vi "Get Ethernet Port.vi"(8 "Error In":errorcluster, 11 "LINX Device Config":T1) -> (0 "Error Out":errorcluster, 2 "Ethernet Port":u16, 3 "LINX Device Config":T1)   [LabVIEW 2020, in "LMH-LINX.lvlib" / "Device.lvlib"]
doc: "Get the LINX device's Ethernet Port."
uses:
  Device.lvlib
  Type Defs/LINX Device Config.ctl
  Type Defs/Interface.ctl
  Type Defs/TCP Config.ctl
  Type Defs/Channels.ctl
  Type Defs/Error Type.ctl
  LMH-LINX.lvlib
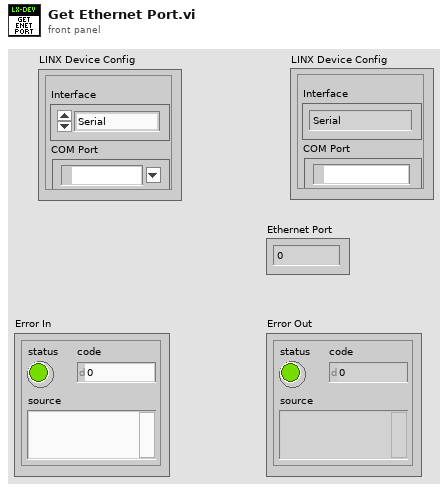
[diagram p1: front panel]
types:
  T1 = typedef "LMH-LINX.lvlib/Device.lvlib/LINX Device Config.ctl" = cluster{"Interface":T2, "COM Port":refnum<visa-resource-name>, "TCP Configuration":T3, "Device Family":u8, "Device ID":u8, "Device Name":string, "TCP Ref":refnum<k5>, "Channels":T4}
  T2 = typedef "LMH-LINX.lvlib/Interface.ctl" = enum16{"Serial", "TCP"}
  T3 = typedef "LMH-LINX.lvlib/Device.lvlib/TCP Config.ctl" = cluster{"IP Address":string, "Port":u16}
  T4 = typedef "LMH-LINX.lvlib/Channels.ctl" = cluster{"DI":u8[], "DO":u8[], "AI":u8[], "AO":u8[], "PWM":u8[], "QE":u8[], "UART":u8[], "I2C 2":u8[], "SPI":u8[], "CAN":u8[], "Servo":u8[], "AI Ref (V)":dbl, "AI Resolution (Bits)":u8, "AO Ref (V)":dbl, "AO Resolution (Bits)":u8}
  T5 = typedef "LMH-LINX.lvlib/Error Type.ctl" = enum16{"Unknown", "Timeout", "Corrupt Return Packet", "Unable To Connect", "Command Not Supported", "Channel DNE", "Invalid COM Config", "Firmware Version Mismatch", "myRIO Support", "CMD Specific Error", "Local IO Not Supported"}
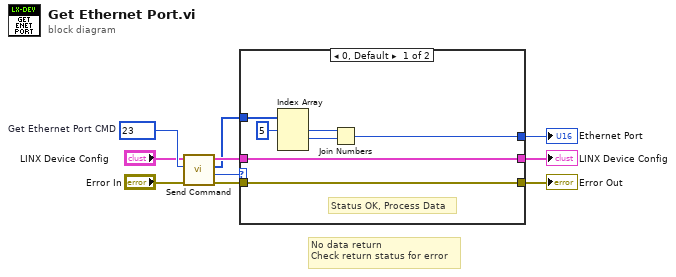
[diagram p0: block diagram]
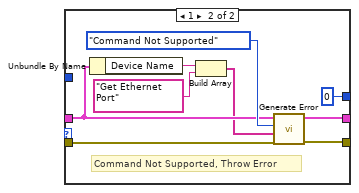
[diagram p2: hidden frame]
diagram:
  w9 = u16 23  # Get Ethernet Port CMD
  # "No data return\nCheck return status for error"
  n1 = call "Send Command.vi"("Error In"="Error In", "CMD"=w9, "LINX Device Config"="LINX Device Config") -> ("Error Out"=w4:errorcluster, "Status"=w1:u8, "Response"=w3:u8[], "LINX Device Config"=w6:T1)  [unwired: 5 in]
  n2 = case shown="0, Default" w1 {
    tunnel: [w16 w24] -> w7
    tunnel: w6 -> [w16 w20]
    tunnel: [w17 w25] -> w5
    tunnel: w4 -> [w17 w26]
    tunnel: w3 -> [w15 _]
    tunnel: [w11 u16 0] -> w2
    frame 0, Default {
      # "Status OK, Process Data"
      n3 = Index Array(array=w15, index #1=5 ("index")) -> (element #1=w13:u8, element #2=w12:u8)  [unwired: 2 in, 1 out]
      n4 = Join Numbers(hi=w13, lo=w12) -> ((hi.lo)=w11:u16)
    }
    frame 1 {
      # "Command Not Supported, Throw Error"
      n5 = Unbundle By Name(w20) -> ("Device Name"=w21:string)
      n6 = Build Array(w21, "Get Ethernet Port") -> (w19:string[])
      n7 = call "Generate Error.vi"("Error In"=w26, "Arguments"=w19, "Error Type"=Error_Type."Command Not Supported", "LINX Device Config"=w20) -> ("Error Out"=w25:errorcluster, "Dup LINX Device Config"=w24:T1)  [unwired: 6 in]
    }
  }
  "Error Out" <- w5
  "LINX Device Config" <- w7
  "Ethernet Port" <- w2
